vi "Read CSM-VI Info.vi"(6 "Config Path":path, 8 "error in (no error)":errorcluster, 11 "CSM Name":string) -> (0 "error out":errorcluster, 3 "Cluster 2":cluster{"Path":path})   [LabVIEW 2017, in "CSM-Helper API with lvcsm Support.lvlib"]
uses:
  CSM-Helper API with lvcsm Support.lvlib
  <vilib>/Utility/config.llb/Read Key (String).vi
  <vilib>/Utility/config.llb/NI_LVConfig.lvlib
  lvcsmFile/lvcsm File Support.lvlib
  _Shared/CSM Shared.lvlib
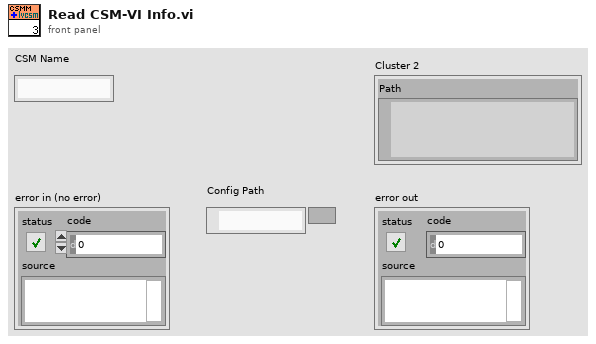
[diagram p1: front panel]
types:
  T1 = typedef "NI_LVConfig.lvlib/Config Data RefNum.ctl" = refnum<k1>
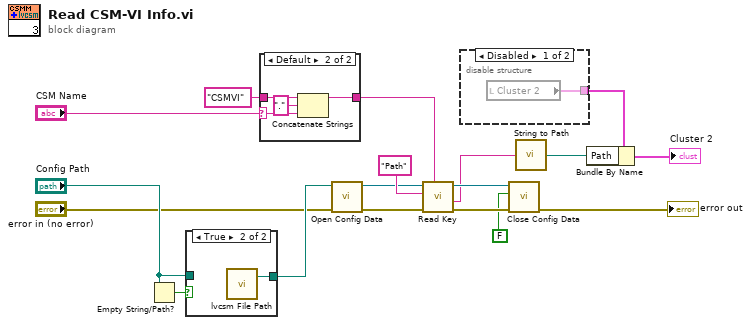
[diagram p0: block diagram]
diagram:
  n1 = Empty String/Path?(string/path="Config Path") -> (empty?=w16:bool)
  n2 = case shown="True" w16 {
    tunnel: [w19 w20] -> w18
    tunnel: "Config Path" -> [w19 _]
    frame False {
    }
    frame True {
      n3 = call "lvcsm File Path.vi"() -> ("Appended Path"=w20:path)  [unwired: 3 in]
    }
  }
  n4 = case shown="Default" "CSM Name" {
    selector: "CSM Name" -> [_ w23]
    tunnel: "CSMVI" ("Section Prefix") -> [w21 w25]
    tunnel: [w21 w24] -> w10
    frame "" {
    }
    frame Default {
      n5 = Concatenate Strings(w25, "." ("string"), w23) -> (w24:string)
    }
  }
  n6 = call <vilib>:"Open Config Data.vi"("error in (no error)"="error in (no error)", "configuration file path"=w18) -> ("error out"=w6:errorcluster, "refnum"=w7:T1)  [unwired: 7 in, 1 out]
  n7 = call-poly <vilib>:"Read Key.vi"("section"=w10, "error in (no error)"=w6, "key"="Path", "refnum"=w7) -> ("error out"=w8:errorcluster, "value"=w3:string, "refnum out"=w9:T1)  [unwired: 4 in, 1 out]
  n8 = disable-structure shown="Disabled" {
    disable-tunnel: [w26 _] -> w4
    frame Disabled {
      n9 = local read "Cluster 2"() -> (w26:cluster{"Path":path})
    }
    frame Enabled {
    }
  }
  n10 = call <vilib>:"Close Config Data.vi"("error in (no error)"=w8, "write file if changed (T)"=FALSE, "refnum"=w9) -> ("error out"=→"error out":errorcluster)  [unwired: 7 in, 1 out]
  n11 = call "String to Path.vi"("String"=w3) -> ("Path"=w1:path)
  n12 = Bundle By Name(cluster=w4, "Path"=w1) -> (→"Cluster 2":cluster{"Path":path})
